vi "autonSample.vi"(0 "Auton Array":dbl[][](array[numeric]), 5 "MeasuredHeading":dbl, 9 "EncoderDistance":dbl) -> (4 "Left Drive":dbl(knob) scale=-1.0..1.0, 6 "Right Drive":dbl(knob) scale=-1.0..1.0, 10 "Turret Rotation":dbl, 14 "Feeder motor":dbl, 15 "Shooter motor output":dbl)   [LabVIEW 2011]
uses:
  Robot Global Data.vi
  <vilib>/addons/control/pid/pid.llb/PID (DBL).vi
  <vilib>/addons/control/pid/NI_PID_pid.lvlib
panel:
  out "Tzero":i64
  out "AccumDist":dbl
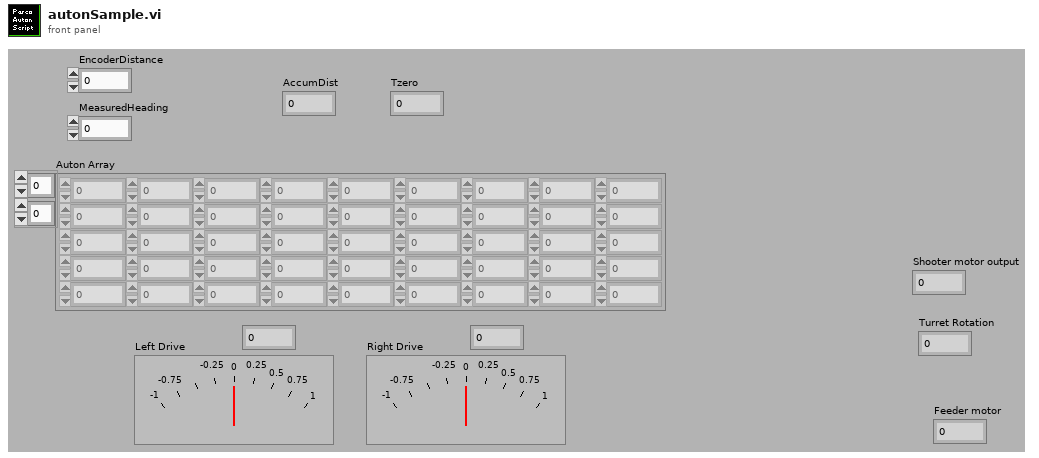
[diagram p1: front panel]
types:
  T1 = cluster{"proportional gain (Kc)":dbl, "integral time (Ti, min)":dbl, "derivative time (Td, min)":dbl}
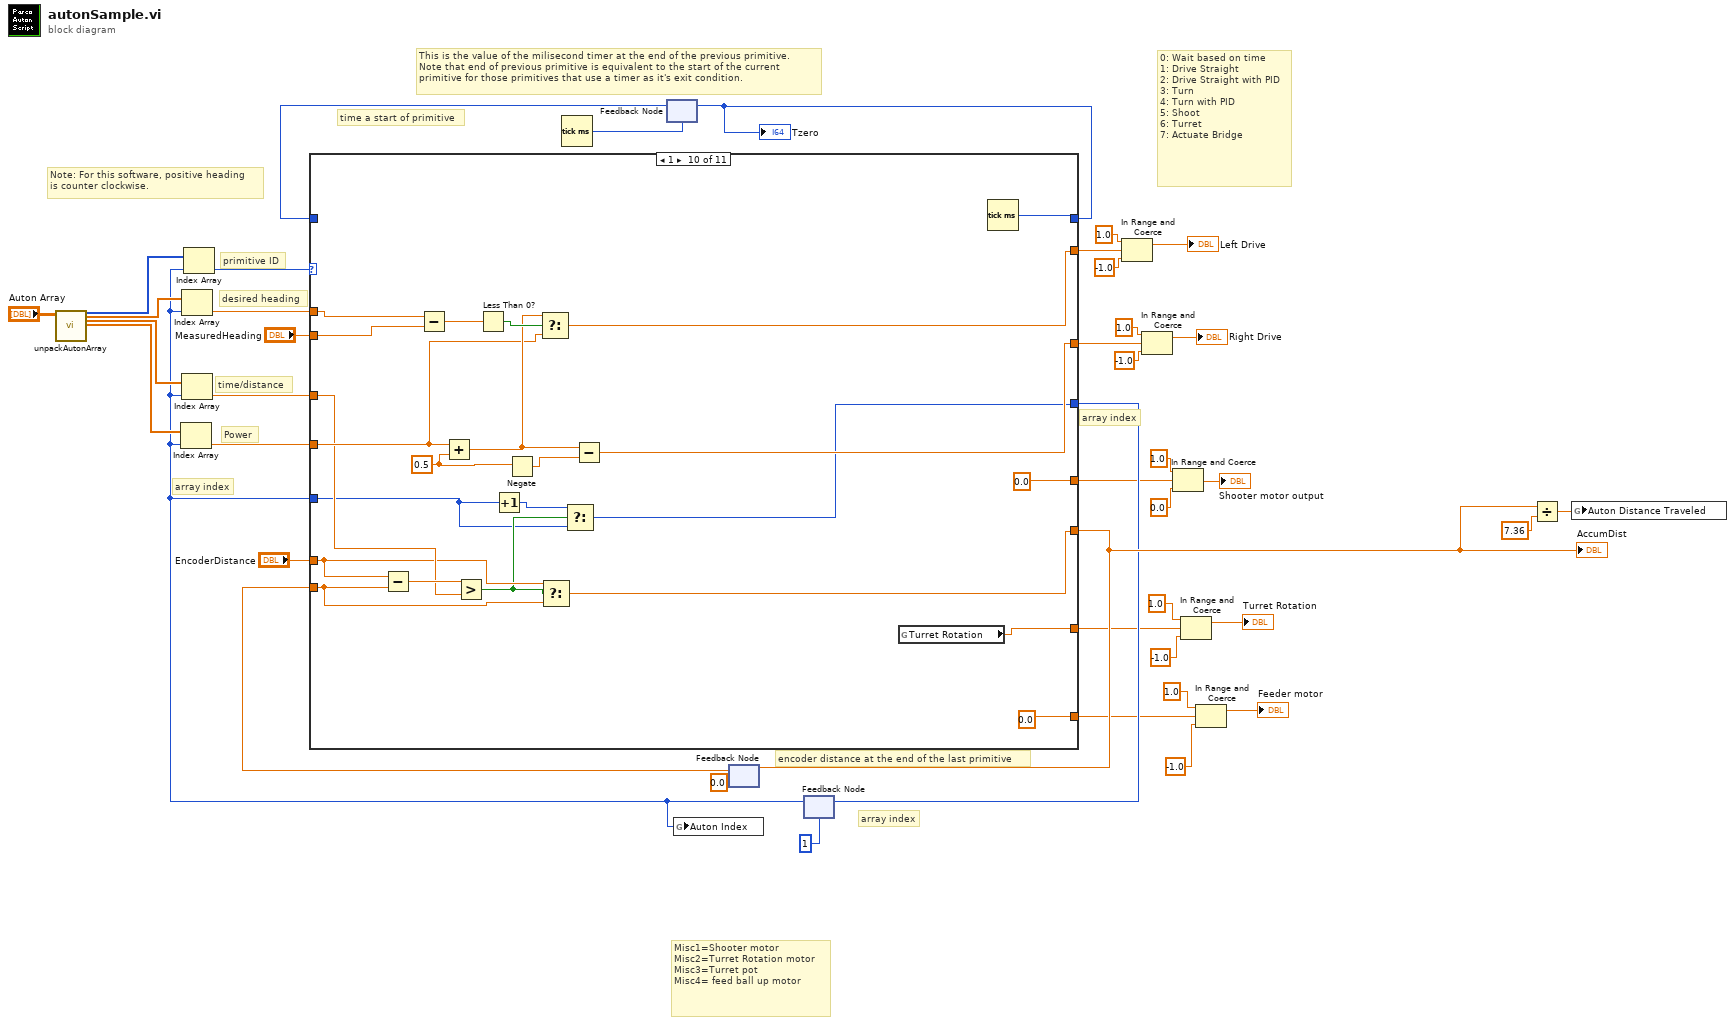
[diagram p0: block diagram]
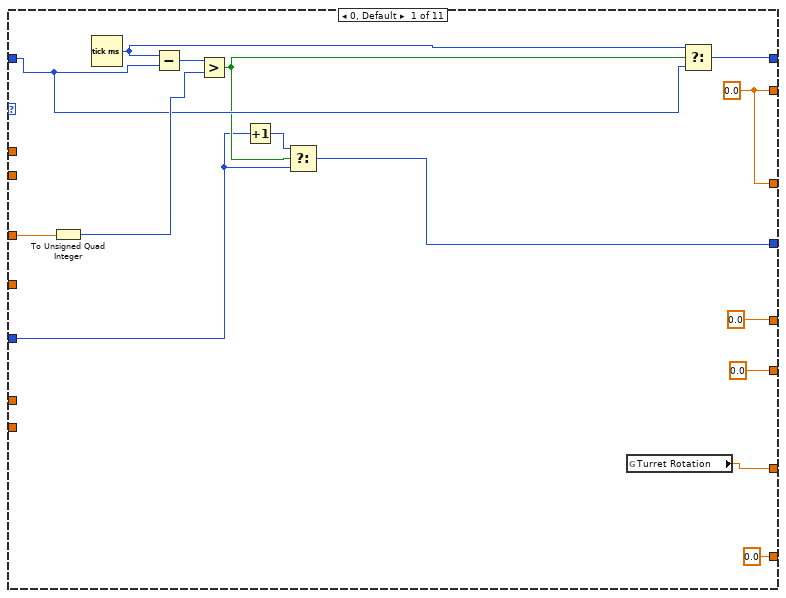
[diagram p2: hidden frame]
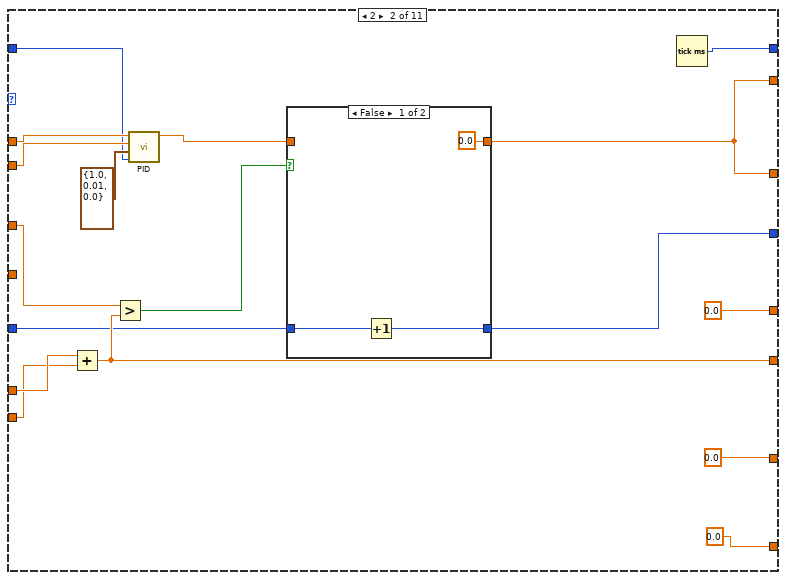
[diagram p3: hidden frame]
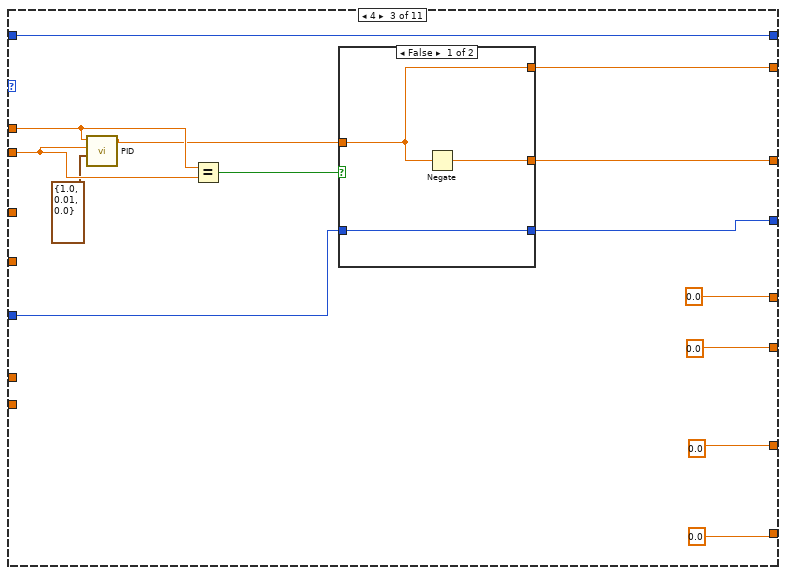
[diagram p5: hidden frame]
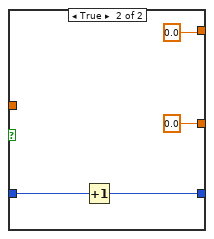
[diagram p6: hidden frame]
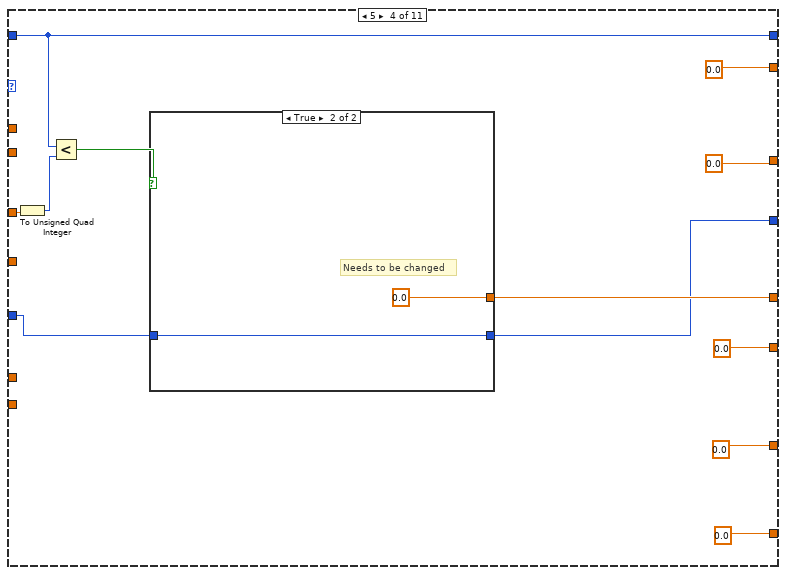
[diagram p7: hidden frame]
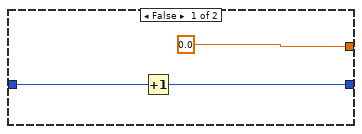
[diagram p8: hidden frame]
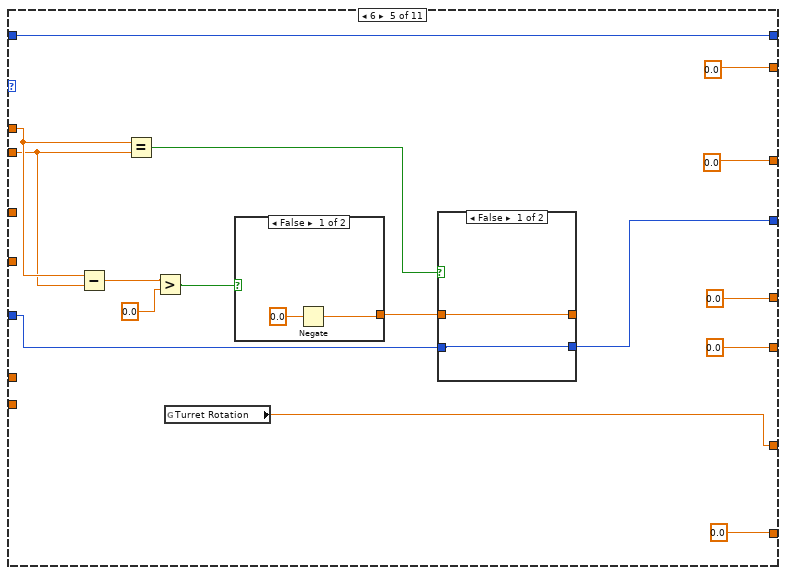
[diagram p9: hidden frame]
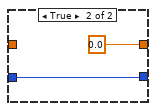
[diagram p10: hidden frame]
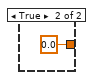
[diagram p11: hidden frame]
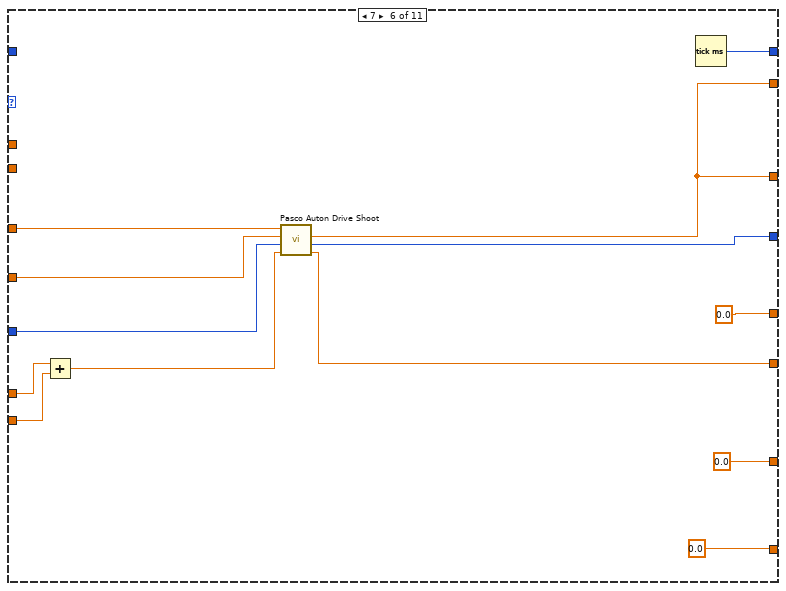
[diagram p12: hidden frame]
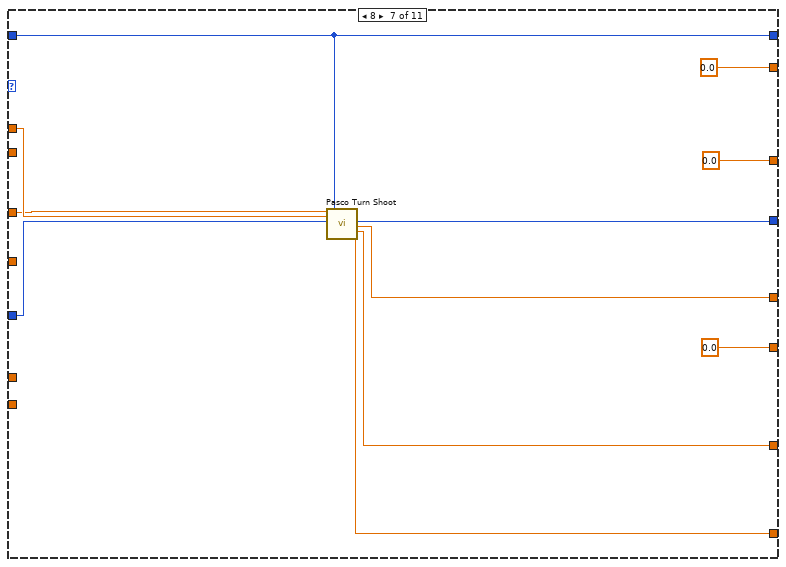
[diagram p13: hidden frame]
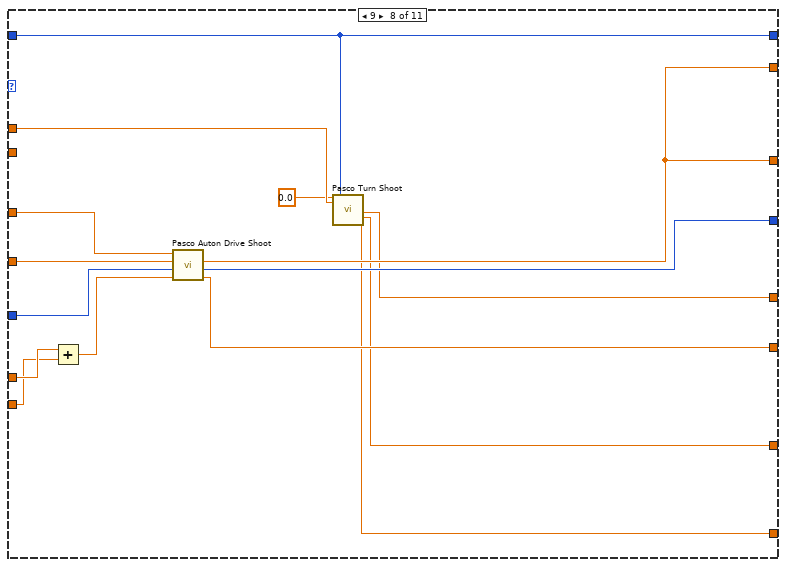
[diagram p14: hidden frame]
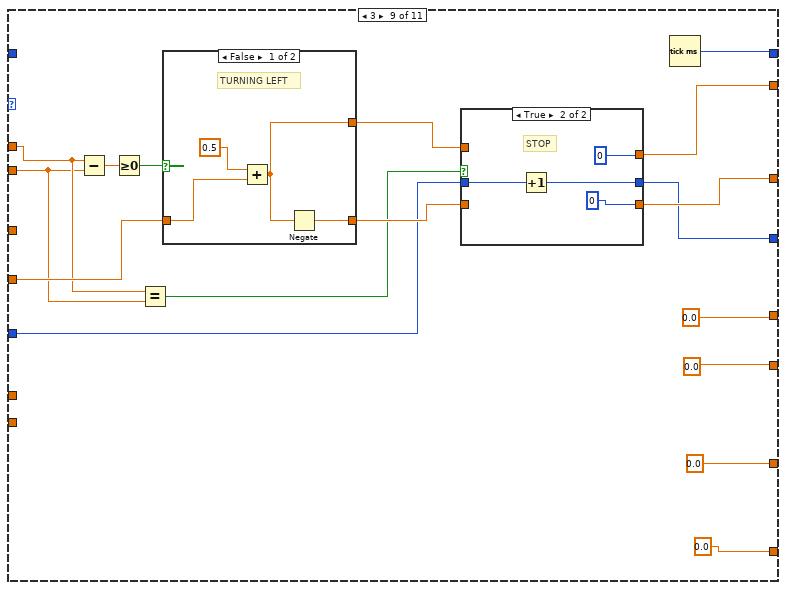
[diagram p15: hidden frame]
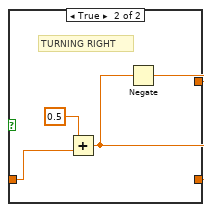
[diagram p17: hidden frame]
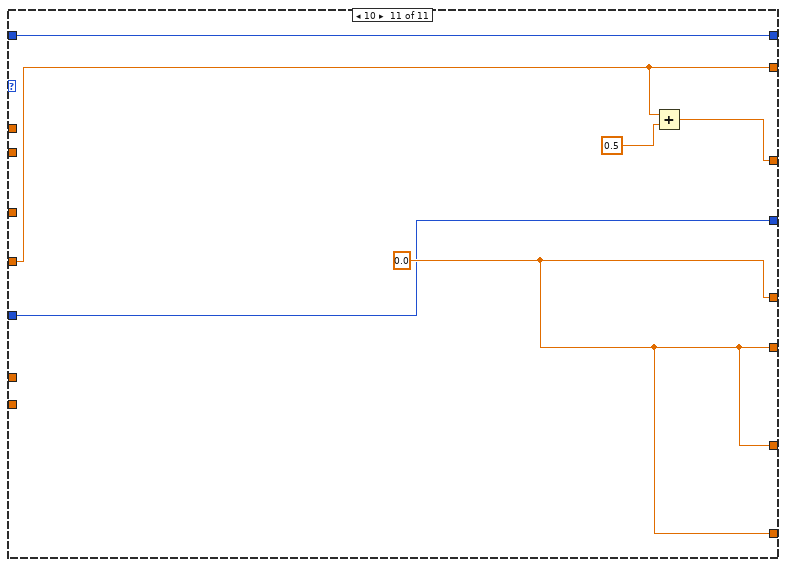
[diagram p18: hidden frame]
diagram:
  # "Misc1=Shooter motor\nMisc2=Turret Rotation motor\nMisc3=Turret pot\nMisc4= feed ball up motor"
  # "0: Wait based on time\n1: Drive Straight\n2: Drive Straight with PID\n3: Turn\n4: Turn with PID\n5: Shoot\n6: Turret\n7: Actuate Bridge"
  # "encoder distance at the end of the last primitive"
  # "Note: For this software, positive heading\nis counter clockwise."
  # "time a start of primitive"
  # "array index"
  # "array index"
  # "This is the value of the milisecond timer at the end of the previous primitive.\nNote that end of previous primitive is equivalent to the start of the current\nprimitive for those primitives that use a timer as it's exit condition."
  # "Power"
  # "array index"
  # "desired heading"
  # "primitive ID"
  # "time/distance"
  n1 = call "unpackAutonArray.vi"("all rows"="Auton Array") -> ("Primitive"=w41:i16[], "Heading"=w23:dbl[], "Distance/Time"=w24:dbl[], "Power"=w21:dbl[])  [unwired: 1 in, 22 out]
  n2 = Tick Count (ms)() -> (millisecond timer value=w35:u32)
  n3 = feedback #1(w35) -> (w39:u32)
  n4 = feedback #2(0.0 ("EncoderDistance")) -> (w20:dbl)
  n5 = feedback #3(1) -> (w2:i32)
  n6 = Index Array(array=w21, index=w2) -> (element=w37:dbl)
  n7 = Index Array(array=w23, index=w2) -> (element=w22:dbl)
  n8 = Index Array(array=w24, index=w2) -> (element=w38:dbl)
  n9 = Index Array(array=w41, index=w2) -> (element=w40:i16)
  n10 = case shown="1" w40 {
    tunnel: [w45 w66 w87 w107 w129 w146 w161 w172 w185 w213 w239] -> w15
    tunnel: w2 -> [w46 w67 w86 w108 w130 w149 w164 w177 w184 w214 w239]
    tunnel: [w57 w74 w93 w102 w128 w142 w162 w167 w191 w212 w238] -> w25
    tunnel: w39 -> [w53 w58 w93 w102 w128 _ w162 w167 _ _ w238]
    tunnel: w38 -> [w55 w70 _ w112 _ w153 w158 w179 _ w221 _]
    tunnel: w22 -> [_ w59 w82 _ w133 _ w163 w171 w193 w232 _]
    tunnel: [w44 w68 w88 0.0 0.0 w147 0.0 w170 w187 w223 w236] -> w33
    tunnel: [w44 w68 w89 0.0 0.0 w147 0.0 w170 w190 w225 w235] -> w26
    tunnel: w37 -> [_ _ _ _ _ w148 _ w178 w195 w224 w236]
    tunnel: "EncoderDistance" -> [_ w73 _ _ _ w152 _ w176 _ w220 _]
    tunnel: "MeasuredHeading" -> [_ w60 w83 _ w119 _ _ _ w192 w231 _]
    tunnel: [0.0 ("Encoder total") w71 0.0 0.0 0.0 w145 0.0 w173 0.0 w217 w240] -> w17
    tunnel: w20 -> [_ w72 _ _ _ w151 _ w175 _ w219 _]
    tunnel: [0.0 ("Misc1  OUT") 0.0 0.0 w109 0.0 0.0 ("Misc1  OUT") w160 w169 0.0 0.0 w240] -> w11
    tunnel: [w43 0.0 0.0 0.0 w118 0.0 ("Misc1  OUT") w159 w168 0.0 w218 w240] -> w7
    tunnel: [0.0 ("Misc4 OUT") 0.0 0.0 0.0 0.0 0.0 w154 w165 0.0 0.0 w240] -> w3
    frame 0, Default {
      w44 = 0.0 ("Numeric")
      n11 = To Unsigned Quad Integer(1:w55) -> (0:w54:u64)
      n12 = Tick Count (ms)() -> (millisecond timer value=w52:u32)
      n13 = Subtract(x=w52, y=w53) -> (x-y=w56:u32)
      n14 = Greater?(x=w56, y=w54) -> (0:w48:bool)
      n15 = Increment(x=w46) -> (x+1=w47:i32)
      n16 = Select(t=w47, s=w48, f=w46) -> (s? t:f=w45:i32)
      n17 = global read "Robot Global Data.vi" "Turret Rotation"() -> (w43:dbl)
      n18 = Select(t=w52, s=w48, f=w53) -> (s? t:f=w57:u32)
    }
    frame 2 {
      n19 = Add(x=w73, y=w72) -> (x+y=w71:dbl)
      n20 = Greater?(x=w70, y=w71) -> (0:w69:bool)
      n21 = call-poly <vilib>:"PID.vi"("dt (s)"=w58, "PID gains"=T1 {"proportional gain (Kc)"=1.0, "integral time (Ti, min)"=0.01, "derivative time (Td, min)"=0.0}, "process variable"=w60, "setpoint"=w59) -> ("output"=w62:dbl)  [unwired: 6 in, 1 out]
      n22 = case shown="False" w69 {
        tunnel: [0.0 w79] -> w68
        tunnel: w62 -> [_ w79]
        tunnel: w67 -> [w77 w78]
        tunnel: [w76 w78] -> w66
        frame False {
          n23 = Increment(x=w77) -> (x+1=w76:i32)
        }
        frame True {
        }
      }
      n24 = Tick Count (ms)() -> (millisecond timer value=w74:u32)
    }
    frame 4 {
      n25 = call-poly <vilib>:"PID.vi"("PID gains"=T1 {"proportional gain (Kc)"=1.0, "integral time (Ti, min)"=0.01, "derivative time (Td, min)"=0.0}, "process variable"=w83, "setpoint"=w82) -> ("output"=w81:dbl)  [unwired: 7 in, 1 out]
      n26 = Equal?(x=w82, y=w83) -> (x = y?=w85:bool)
      n27 = case shown="False" w85 {
        tunnel: w81 -> [w95 _]
        tunnel: [w96 0.0] -> w89
        tunnel: [w95 0.0] -> w88
        tunnel: [w94 w99] -> w87
        tunnel: w86 -> [w94 w100]
        frame False {
          n28 = Negate(x=w95) -> (-x=w96:dbl)
        }
        frame True {
          n29 = Increment(x=w100) -> (x+1=w99:i32)
        }
      }
    }
    frame 5 {
      n30 = To Unsigned Quad Integer(1:w112) -> (0:w110:u64)
      n31 = Less?(x=w102, y=w110) -> (x < y?=w111:bool)
      n32 = case shown="True" w111 {
        tunnel: [0.0 0.0] -> w109
        tunnel: w108 -> [w114 w117]
        tunnel: [w113 w117] -> w107
        frame False {
          n33 = Increment(x=w114) -> (x+1=w113:i32)
        }
        frame True {
          # "Needs to be changed"
        }
      }
    }
    frame 6 {
      n34 = Subtract(x=w133, y=w119) -> (x-y=w121:dbl)
      n35 = Equal?(x=w133, y=w119) -> (x = y?=w132:bool)
      n36 = Greater?(x=w121, y=0.0) -> (0:w122:bool)
      n37 = global read "Robot Global Data.vi" "Turret Rotation"() -> (w118:dbl)
      n38 = case shown="False" w122 {
        tunnel: [w139 0.0] -> w131
        frame False {
          n39 = Negate(x=0.0) -> (-x=w139:dbl)
        }
        frame True {
        }
      }
      n40 = case shown="False" w132 {
        tunnel: [w135 0.0] -> _
        tunnel: w131 -> [w135 _]
        tunnel: w130 -> [w134 w137]
        tunnel: [w134 w137] -> w129
        frame False {
        }
        frame True {
        }
      }
    }
    frame 7 {
      n41 = Add(x=w152, y=w151) -> (x+y=w150:dbl)
      n42 = call "Pasco Auton Drive Shoot.vi"("Encoder total"=w150, "Array"=w149, "Power"=w148, "time/distance"=w153) -> ("Encoder total"=w145:dbl, "Array Out"=w146:i32, "Power"=w147:dbl)  [unwired: 5 in]
      n43 = Tick Count (ms)() -> (millisecond timer value=w142:u32)
    }
    frame 8 {
      n44 = call "Pasco Turn Shoot.vi"("time/distance"=w158, "desired heading"=w163, "array index"=w164, "primitive time"=w162) -> ("array index"=w161:i32, "Misc1  OUT"=w160:dbl, "Misc2 OUT"=w159:dbl, "Misc4 OUT"=w154:dbl)  [unwired: 12 in]
    }
    frame 9 {
      n45 = Add(x=w176, y=w175) -> (x+y=w174:dbl)
      n46 = call "Pasco Auton Drive Shoot.vi"("Encoder total"=w174, "Array"=w177, "Power"=w178, "time/distance"=w179) -> ("Encoder total"=w173:dbl, "Array Out"=w172:i32, "Power"=w170:dbl)  [unwired: 5 in]
      n47 = call "Pasco Turn Shoot.vi"("time/distance"=0.0, "desired heading"=w171, "primitive time"=w167) -> ("Misc1  OUT"=w169:dbl, "Misc2 OUT"=w168:dbl, "Misc4 OUT"=w165:dbl)  [unwired: 13 in, 1 out]
    }
    frame 3 {
      n48 = Subtract(x=w193, y=w192) -> (x-y=w196:dbl)
      n49 = Greater Or Equal To 0?(x=w196) -> (x >= 0?=w194:bool)
      n50 = Equal?(x=w193, y=w192) -> (x = y?=w186:bool)
      n51 = case shown="False" w194 {
        tunnel: w195 -> [w206 w208]
        tunnel: [w204 w210] -> w188
        tunnel: [w205 w209] -> w189
        frame False {
          # "TURNING LEFT"
          n52 = Add(x=0.5, y=w206) -> (x+y=w204:dbl)
          n53 = Negate(x=w204) -> (-x=w205:dbl)
        }
        frame True {
          # "TURNING RIGHT"
          n54 = Add(x=0.5, y=w208) -> (x+y=w209:dbl)
          n55 = Negate(x=w209) -> (-x=w210:dbl)
        }
      }
      n56 = case shown="True" w186 {
        tunnel: w184 -> [w199 w203]
        tunnel: [w199 w202] -> w185
        tunnel: [w198 0] -> w190
        tunnel: w189 -> [w198 _]
        tunnel: [w197 0] -> w187
        tunnel: w188 -> [w197 _]
        frame False {
          # "DRIVE"
        }
        frame True {
          # "STOP"
          n57 = Increment(x=w203) -> (x+1=w202:i32)
        }
      }
      n58 = Tick Count (ms)() -> (millisecond timer value=w191:u32)
    }
    frame 1 {
      w227 = 0.5 ("y")
      n59 = Subtract(x=w220, y=w219) -> (x-y=w222:dbl)
      n60 = Subtract(x=w232, y=w231) -> (x-y=w230:dbl)
      n61 = Add(x=w224, y=w227) -> (x+y=w228:dbl)
      n62 = Greater?(x=w222, y=w221) -> (0:w216:bool)
      n63 = Less Than 0?(x=w230) -> (x < 0?=w229:bool)
      n64 = Increment(x=w214) -> (x+1=w215:i32)
      n65 = Negate(x=w227) -> (-x=w226:dbl)
      n66 = Select(t=w228, s=w229, f=w224) -> (s? t:f=w223:dbl)
      n67 = Select(t=w220, s=w216, f=w219) -> (s? t:f=w217:dbl)
      n68 = Select(t=w215, s=w216, f=w214) -> (s? t:f=w213:i32)
      n69 = Subtract(x=w228, y=w226) -> (x-y=w225:dbl)
      n70 = global read "Robot Global Data.vi" "Turret Rotation"() -> (w218:dbl)
      n71 = Tick Count (ms)() -> (millisecond timer value=w212:u32)
    }
    frame 10 {
      w240 = 0.0
      n72 = Add(x=w236, y=0.5 ("x+y")) -> (x+y=w235:dbl)
    }
  }
  "AccumDist" <- w17
  "Tzero" <- w25
  n73 = feedback-in #1(w25) -> ()
  n74 = global write "Robot Global Data.vi" "Auton Index"(w2) -> ()
  n75 = feedback-in #2(w17) -> ()
  n76 = feedback-in #3(w15) -> ()
  n77 = In Range and Coerce(upper limit=1.0, x=w33, lower limit=-1.0) -> (coerced(x)=→"Left Drive":dbl)  [unwired: 1 out]
  n78 = In Range and Coerce(upper limit=1.0, x=w26, lower limit=-1.0) -> (coerced(x)=→"Right Drive":dbl)  [unwired: 1 out]
  n79 = In Range and Coerce(upper limit=1.0, x=w11, lower limit=0.0) -> (coerced(x)=→"Shooter motor output":dbl)  [unwired: 1 out]
  n80 = In Range and Coerce(upper limit=1.0, x=w7, lower limit=-1.0) -> (coerced(x)=→"Turret Rotation":dbl)  [unwired: 1 out]
  n81 = In Range and Coerce(upper limit=1.0, x=w3, lower limit=-1.0) -> (coerced(x)=→"Feeder motor":dbl)  [unwired: 1 out]
  n82 = Divide(x=w17, y=7.36) -> (x/y=w1:dbl)
  n83 = global write "Robot Global Data.vi" "Auton Distance Traveled"(w1) -> ()
